vi "absCalcPlot.vi"   [LabVIEW 2011]
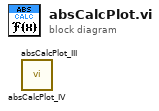
[diagram p0: block diagram]
diagram:
  n1 = call "absCalcPlot_IV.vi"() -> ()  [unwired: 8 in, 4 out]
  n2 = call "absCalcPlot_III.vi"() -> ()  [unwired: 8 in, 4 out]
